vi "TUNA hindbrain ACT.vi"(4 "Manual?":bool=TRUE, 6 "error in":errorcluster, 7 "Act Com":T1, 8 "MHeading":dbl(slide) scale=0.0005..0.0025 scale format="%_1f", 9 "MSpeed":dbl(slide) scale=0.0005..0.0025 scale format="%#.1g") -> (0 "error out":errorcluster, 1 "Speed":dbl min=-9.0 max=9.0 step=1.0, 2 "Rudder":dbl min=-45.0 max=45.0 step=1.0, 3 "Desired\nSpeed":dbl, 5 "Desired \nRudder":dbl)   [LabVIEW 2014]
doc: "This vi has two functions: it selects between manual and auto mode and it converts the incoming value into speed and rudder control values."
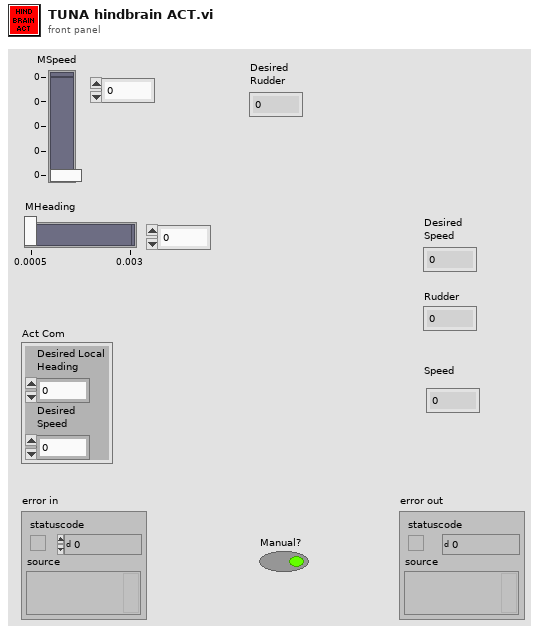
[diagram p1: front panel]
types:
  T1 = cluster{"Desired Local\nHeading":dbl, "Desired\nSpeed":dbl}
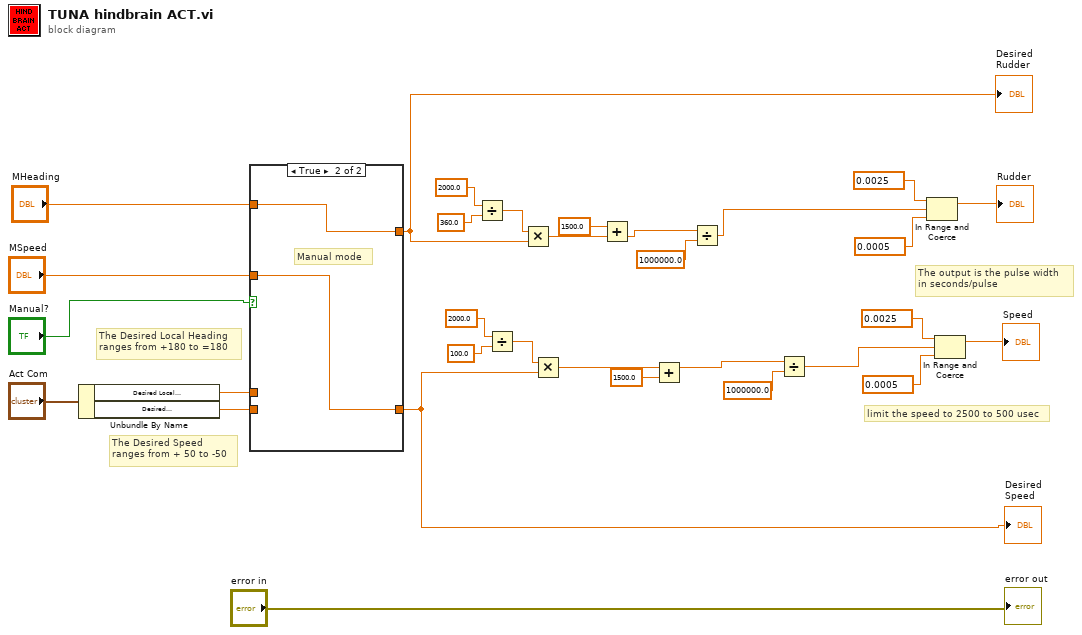
[diagram p0: block diagram]
diagram:
  # "The output is the pulse width\nin seconds/pulse"
  # "The Desired Local Heading\nranges from +180 to =180"
  # "The Desired Speed\nranges from + 50 to -50"
  # "limit the speed to 2500 to 500 usec"
  n1 = Unbundle By Name("Act Com") -> ("Desired Local\nHeading"=w23:dbl, "Desired\nSpeed"=w22:dbl)
  n2 = case shown="True" "Manual?" {
    tunnel: w23 -> [w33 _]
    tunnel: [w33 w35] -> w15
    tunnel: w22 -> [w32 _]
    tunnel: [w32 w34] -> w6
    tunnel: "MHeading" -> [_ w35]
    tunnel: "MSpeed" -> [_ w34]
    frame False {
      # "Auto mode"
    }
    frame True {
      # "Manual mode"
    }
  }
  "Desired \nRudder" <- w15
  "Desired\nSpeed" <- w6
  n3 = Divide(x=2000.0, y=360.0) -> (x/y=w16:dbl)
  n4 = Divide(x=2000.0, y=100.0) -> (x/y=w9:dbl)
  n5 = Multiply(x=w16, y=w15) -> (x*y=w14:dbl)
  n6 = Multiply(x=w9, y=w6) -> (x*y=w8:dbl)
  n7 = Add(x=1500.0, y=w14) -> (x+y=w4:dbl)
  n8 = Add(x=w8, y=1500.0) -> (x+y=w2:dbl)
  n9 = Divide(x=w4, y=1000000.0) -> (x/y=w12:dbl)
  n10 = Divide(x=w2, y=1000000.0) -> (x/y=w5:dbl)
  n11 = In Range and Coerce(upper limit=0.0025 ("t"), x=w12, lower limit=0.0005 ("t")) -> (coerced(x)=→"Rudder":dbl)  [unwired: 1 out]
  n12 = In Range and Coerce(upper limit=0.0025 ("t"), x=w5, lower limit=0.0005 ("t")) -> (coerced(x)=→"Speed":dbl)  [unwired: 1 out]
  "error out" <- "error in"
